vi "Tosca-Test New Schedule.vi"() -> ()   [LabVIEW 2015]
panel:
  in  "Path":path=path "C:/Data/Tosca/Parameters/test.ini"
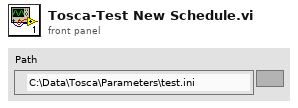
[diagram p1: front panel]
types:
  T1 = typedef "Tosca-Parameters.ctl" = cluster{"Description":string, "Output States":T2, "Input Events":T34[], "Flowchart":T38[], "DAQ":T43, "Masker":T45, "Imaging":T46, "Adapt":T48, "MATLAB function":path, "Schedule":T52, "Pretrial":T58, "AI":T59, "ParamFile":path, "Flags":T60[]}
  T2 = typedef "Output State Array.xctl/Data.ctl" = T3[]
  T3 = typedef "Single Output State.ctl" = cluster{"Name":string, "T (s)":dbl, "StimChans":T4, "First AO":dbl[][], "Npoll":i32, "Continue?":bool, "Max Nrep":i32, "First DO":bool[][], "AO":T30, "DO":T31, "immediate":bool, "Grating":T32}
  T4 = typedef "Multichannel (Full).xctl/Data.ctl" = T5[]
  T5 = typedef "Stimulus Channel (Full).xctl/Full Stimulus Channel Data.ctl" = cluster{"Waveform":T6, "Filter":T23, "Burst":T25, "Level":T26, "Name":string, "Advanced":T28, "SAM":T29}
  T6 = typedef "Waveform XCtl.xctl/Waveform Data.ctl" = cluster{"Type":T7, "Tone":T8, "Pulse Train":T9, "Noise":T12, "File":T13, "FMSweep":T14, "Chirp Train":T15, "Complex Tone":cluster{"Params":T17, "Data":T19}, "Moving Ripple":T20}
  T7 = typedef "Waveform Enum.ctl" = enum16{"OFF", "Tone", "Noise", "Pulse Train", "File", "FM Sweep", "Chirp Train", "Complex Tone", "FM Tone", "Moving Ripple"}
  T8 = typedef "Tone Params.ctl" = cluster{"Frequency (kHz)":dbl, "Last Freq":dbl, "Last Phase":dbl}
  T9 = typedef "Pulse Train Params.ctl" = cluster{"Pulse width (us)":dbl, "Pulse rate (Hz)":dbl, "Gap (ms)":dbl, "Polarity":T10, "PT State":T11, "Asynch":bool}
  T10 = typedef "Pulse Polarity.ctl" = enum16{"POS", "NEG", "POS-NEG", "NEG-POS"}
  T11 = typedef "PT-Continuous State.ctl" = cluster{"Template":dbl[], "Nperiod":i32, "Index":i32, "Pulse Rate (Hz)":dbl, "Phase (cycles)":dbl, "Noff":i32}
  T12 = typedef "Noise Params.ctl" = cluster{"InvFilt":bool, "Noise":dbl[], "CurPt":i32, "Aweight":bool, "Seed":i32, "afile":path}
  T13 = typedef "StimFile-Params.ctl" = cluster{"Filename":path, "Signal":dbl[], "Channel":i32, "stream":bool, "offset":i32, "nreps":i32}
  T14 = typedef "FM Sweep Params.ctl" = cluster{"Rate (oct/s)":dbl, "Fmin (Hz)":dbl, "Fmax (Hz)":dbl, "Ramp (ms)":dbl, "Linear":bool}
  T15 = typedef "Chirp Train.ctl" = cluster{"Params":T16, "Data":cluster{"WF":dbl[]}}
  T16 = typedef "Chirp Train Params.ctl" = cluster{"Fmin (kHz)":dbl, "Fmax (kHz)":dbl, "Compensate":bool, "Duration (ms)":dbl}
  T17 = typedef "CT-Params.ctl" = cluster{"F0 (Hz)":dbl, "Band":cluster{"Flow (Hz)":dbl, "Fhigh (Hz)":dbl}, "Phase":T18, "Min F0 (Hz)":dbl, "Max F0 (Hz)":dbl, "ContinRandPhase":bool, "Max peak factor":dbl, "Max mod depth":dbl, "MinHarmNum":i32, "MaxHarmNum":i32, "Level Mode":enum16{"per component", "overall rms"}, "% jitter":dbl}
  T18 = typedef "CT-Phase Enum.ctl" = enum16{"Cosine", "Random", "Alternating"}
  T19 = typedef "CT-Runtime Data.ctl" = cluster{"Ncomp":i32, "MinHarm":i32, "Phase":dbl[], "Amplitude":dbl[], "Npts/frame":i32, "Last F0":dbl, "Fmin":dbl, "Fmax":dbl, "Lslope":dbl, "randphase":bool, "overall rms":bool, "fmult":dbl[], "jittered":bool}
  T20 = typedef "Moving Ripple.ctl" = cluster{"Params":T21, "Data":T22}
  T21 = typedef "Moving Ripple.Params.ctl" = cluster{"Fmin":dbl, "Fmax":dbl, "Density":dbl, "Velocity":dbl, "Depth":dbl, "Phase":dbl, "Comp/oct":i32}
  T22 = typedef "Moving Ripple.Data.ctl" = cluster{"Components":dbl[]}
  T23 = typedef "Advanced Filter XCtl.xctl/Filter Data.ctl" = cluster{"Type":enum16{"Lowpass", "Highpass", "Bandpass", "Bandstop", "OFF"}, "CF (kHz)":dbl, "BW (kHz)":dbl, "Cascade":bool, "Quadrature":bool, "Scale Factor":dbl, "Stages":cluster{"IIR Filter":cluster{"filter structure":enum32{"IIR 2nd Order", "IIR 4th Order"}, "Reverse Coefficients":dbl[], "Forward Coefficients":dbl[]}, "State":dbl[]}[], "Class":enum16{"Elliptic", "Butterworth"}, "Order":i32, "BWUnits":T24}
  T24 = typedef "Filter-Bandwidth Units.ctl" = enum16{"Linear", "Octaves", "Min-Max"}
  T25 = typedef "Burst Control.xctl/Burst Data.ctl" = cluster{"Active":bool, "Delay (ms)":dbl, "Duration (ms)":dbl, "Ramp (ms)":dbl, "Rate (Hz)":dbl, "Trepeat (ms)":dbl, "Repeat":bool}
  T26 = typedef "Level XCtl.xctl/Level Data.ctl" = cluster{"Level":dbl, "Units":T27, "Max":dbl, "Multiplier":dbl, "Cal File":path, "Cal":cluster{"Freq (Hz)":dbl[], "Mag (dB SPL)":dbl[], "Phase (deg)":dbl[]}}
  T27 = typedef "Level Units.ctl" = enum16{"dB atten", "dB SPL", "dB re 1 Vrms", "dB V/Hz½", "mW", "dB HL", "Volts", "dB mW"}
  T28 = typedef "Advanced Stimulus Options.xctl/Advanced Stimulus Options.ctl" = cluster{"Rep Mask":string, "AltPol":bool, "Var":string, "Expr":string, "Persist":bool}
  T29 = typedef "SAM Params.ctl" = cluster{"Active":bool, "Frequency (Hz)":dbl, "Depth":dbl, "Init Phase (cycles)":dbl, "phase (degrees)":dbl, "Asynch":bool}
  T30 = typedef "Tosca-AO Runtime.ctl" = cluster{"Fs (Hz)":dbl, "pts/poll":i32, "pts/rep":i32, "ramp off":bool[], "ledIndex":i32}
  T31 = typedef "Tosca-DO Runtime.ctl" = cluster{"Fs (Hz)":dbl, "pts/poll":i32, "pts/rep":i32, "Rep":i32, "State":i32, "Trial":i32, "Frame":i32, "frOut":bool[], "Nchan":i32}
  T32 = typedef "Tosca-Grating.ctl" = cluster{"Type":T33, "Orientation (deg)":dbl, "Spatial frequency (cpd)":dbl, "Velocity (Hz)":dbl, "Contrast":dbl, "Background intensity":dbl, "Duration (ms)":dbl, "Phase (cycles)":dbl}
  T33 = typedef "Tosca-Grating Type.ctl" = enum16{"OFF", "Square", "Sine"}
  T34 = typedef "Tosca-Input Event.ctl" = cluster{"Name":string, "Criteria":T35[], "Operators":enum16{"AND", "OR"}[], "Accumulator":T37}
  T35 = typedef "Tosca-Input Criterion.ctl" = cluster{"DigInput":i32, "State":T36, "Time (ms)":i32, "Name":string}
  T36 = typedef "Logic State.ctl" = enum16{"Low", "High", "Rising", "Falling"}
  T37 = typedef "Tosca-Accumulator.ctl" = cluster{"active":bool, "N":i32, "T":dbl, "Imax":dbl, "latency":dbl}
  T38 = typedef "Tosca-Flow Element.ctl" = cluster{"Name":string, "State Index":i32, "Row":dbl, "Color":u32, "Selected?":bool, "Timeouts":T39[], "Term Cond":T41[], "rect":cluster{"left":i16, "top":i16, "right":i16, "bottom":i16}, "Target?":bool, "Links":cluster{"forward":i32[], "backward":i32[]}}
  T39 = typedef "Tosca-Timeout Spec.ctl" = cluster{"Next":i32, "rect":cluster{"left":i16, "top":i16, "right":i16, "bottom":i16}, "Row":dbl, "Selected?":bool, "Type":T40, "Units":enum16{"Reps", "Seconds"}, "Expr":string, "TTL":refnum<class "TTLController.lvclass">[]}
  T40 = typedef "Tosca-Event Type.ctl" = enum16{"Normal", "CS+", "CS-"}
  T41 = typedef "Tosca-Termination Condition.ctl" = cluster{"Name":string, "Input Event":i32, "Next":i32, "rect":cluster{"left":i16, "top":i16, "right":i16, "bottom":i16}, "Row":dbl, "Selected?":bool, "Type":T40, "End after (ms)":dbl, "End on rep":bool, "Latency (ms)":dbl, "TTL":refnum<class "TTLController.lvclass">[], "Action":T42, "Nttl":i32, "Tttl":string, "one shot":bool}
  T42 = typedef "Tosca-Termination Condition Action.ctl" = enum16{"End state", "Complete state", "TTL only"}
  T43 = typedef "Tosca-DAQ Options.ctl" = cluster{"AO Sampling Rate (Hz)":dbl, "Poll Rate (Hz)":dbl, "DO Sampling Rate (Hz)":dbl, "Tracking":bool, "Synapse":bool, "Pupil":T44, "Loco":bool, "Retrieve":bool}
  T44 = typedef "Tosca-Pupillometry Mode.ctl" = enum16{"OFF", "EPL", "ETMobile"}
  T45 = typedef "Tosca-Masker Params.ctl" = cluster{"Channel":string}
  T46 = typedef "Tosca-Imaging.ctl" = cluster{"mode":T47, "FrameRateHz":dbl, "LED":string, "Min frames":i32}
  T47 = typedef "Tosca-Imaging Mode.ctl" = enum16{"Off", "Widefield", "Two-photon"}
  T48 = typedef "Tosca-Adapt.ctl" = cluster{"Switch after":i32, "Switch type":enum16{"Trials", "Reversals"}, "Tracks":T49[]}
  T49 = typedef "Tosca-Adaptive Track.ctl" = cluster{"state":string, "chan":string, "param":string, "Start":dbl, "Step":string, "Mode":enum16{"Add", "Multiply"}, "Pcatch":dbl, "Ndown":i32, "Nup":i32, "Nreverse":i32, "Min":dbl, "Max":dbl, "Catch":T50[], "do all catch":bool, "name":string, "Vars":T50[], "compute":T51, "of last":i32, "Step2":string, "after":i32}
  T50 = typedef "Tosca-Simple Variable.ctl" = cluster{"state":string, "chan":string, "param":string, "expr":string}
  T51 = typedef "Tosca-Adapt Threshold Metric.ctl" = enum16{"mean", "median"}
  T52 = typedef "Tosca-Schedule.ctl" = cluster{"Mode":T53, "Blocks":i32, "Decision State":string, "order":T54, "balance":bool, "Families":T55[], "herald":bool}
  T53 = typedef "Tosca-Schedule Mode.ctl" = enum16{"Seq", "CS+/CS-", "Adapt"}
  T54 = typedef "Tosca-Sequence Order.ctl" = enum16{"Sequential", "Alternate", "Randomize", "Random group"}
  T55 = typedef "Tosca-Parameter Family.ctl" = cluster{"Name":string, "Number":i32, "Vars":T56[], "Mask":bool[][], "one each":bool}
  T56 = typedef "Tosca-Parameter Table Element.ctl" = cluster{"state":string, "chan":string, "param":string, "expr":string, "dim":T57, "value":dbl[]}
  T57 = typedef "Tosca-Parameter Dimension.ctl" = enum16{"Ind", "X", "Y"}
  T58 = typedef "Tosca-Pretrial Spec.ctl" = cluster{"Path":path, "Args":string[]}
  T59 = typedef "Tosca-AI.ctl" = cluster{"active":bool, "Fs":dbl, "AI":string[], "DI":string[]}
  T60 = typedef "Tosca-Flag.ctl" = cluster{"Name":string, "Default":i32}
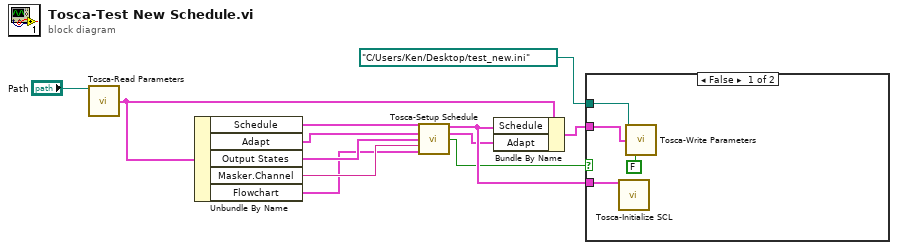
[diagram p0: block diagram]
diagram:
  n1 = call "Tosca-Read Parameters.vi"("Path in"="Path") -> ("Tosca"=w8:T1)  [unwired: 11 in, 3 out]
  n2 = Unbundle By Name(w8) -> ("Schedule"=w11:T52, "Adapt"=w4:T48, "Output States"=w10:T2, "Masker.Channel"=w9:string, "Flowchart"=w1:T38[])
  n3 = call "Tosca-Setup Schedule.vi"("Schedule in"=w11, "Adapt in"=w4, "Output States"=w10, "Masker Channel"=w9, "Pretrial"=w1) -> ("Schedule out"=w5:T52, "Adapt out"=w2:T48, "Canceled?"=w3:bool)  [unwired: 8 in]
  n4 = Bundle By Name(cluster=w8, "Schedule"=w5, "Adapt"=w2) -> (w7:T1)
  n5 = case shown="False" w3 {
    tunnel: w7 -> [w15 _]
    tunnel: path "C:/Users/Ken/Desktop/test_new.ini" ("Path (dialog)") -> [w16 _]
    tunnel: w5 -> [w14 _]
    frame False {
      n6 = call "Tosca-Initialize SCL.vi"("Schedule"=w14) -> ()  [unwired: 13 in, 2 out]
      n7 = call "Tosca-Write Parameters.vi"("Path in"=w16, "Tosca"=w15, "Prompt (T)"=FALSE) -> ()  [unwired: 10 in, 3 out]
    }
    frame True {
    }
  }
